vi "Command2Temp.vi"(10 "DataIn":u8[](array[numeric])) -> (2 "Temp":u8)   [LabVIEW 2013]
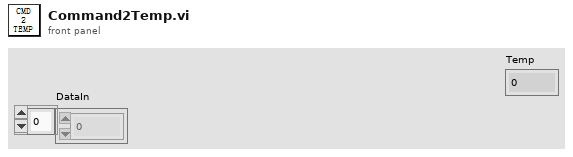
[diagram p1: front panel]
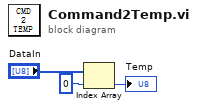
[diagram p0: block diagram]
diagram:
  n1 = Index Array(array="DataIn", index=0) -> (element=→"Temp":u8)
